vi "KH TURCK ETHERNETIP RFID Write data.vi"(8 "Nr RFID":i32, 11 "Channel":u16) -> (3 "Write Data":u8[](array[numeric]))   [LabVIEW 2021]
uses:
  KH TURCK TypeDefs FGlob.ctl
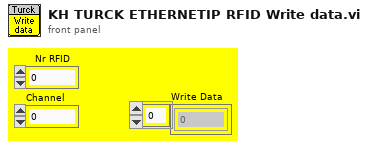
[diagram p1: front panel]
types:
  T1 = typedef "KH TURCK TypeDefs FGlob.ctl" = enum16{"Put one", "Put all", "Recall one", "Recall all"}
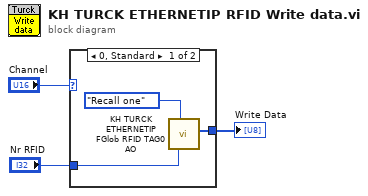
[diagram p0: block diagram]
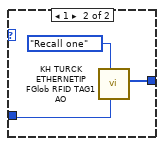
[diagram p2: hidden frame]
diagram:
  n1 = case shown="0, Standard" "Channel" {
    tunnel: [w5 w9] -> w2
    tunnel: "Nr RFID" -> [w4 w7]
    frame 0, Default {
      n2 = call "KH TURCK ETHERNETIP FGlob RFID TAG0 AO.vi"("Nr Module"=w4, "Function"=KH_TURCK_TypeDefs_FGlob."Recall one") -> ("RFID one out"=w5:u8[])  [unwired: 7 in, 2 out]
    }
    frame 1 {
      n3 = call "KH TURCK ETHERNETIP FGlob RFID TAG1 AO.vi"("Nr Module"=w7, "Function"=KH_TURCK_TypeDefs_FGlob."Recall one") -> ("RFID one out"=w9:u8[])  [unwired: 7 in, 2 out]
    }
  }
  "Write Data" <- w2
